vi "test b-field many sesnors tx ty derivatives.vi"() -> ()   [LabVIEW 2017]
uses:
  typedefs/magnet location tx ty.ctl
  typedefs/magnetomter reading set.ctl
panel:
  in  "magnet location tx ty BrV":T1={"x magnet"=20.0, "y magnet"=10.0, "z magnet"=100.0, "tx"=0.0, "ty"=0.0, "BrV"=-990.802948176856}
  out "size(s) 2":i32[](array[numeric])
  out "size(s)":i32[](array[numeric])
  out "derivatives":dbl[][](array[numeric]) format="%#_2p"
  out "numeric derivatives":dbl[][](array[numeric]) format="%#_2p"
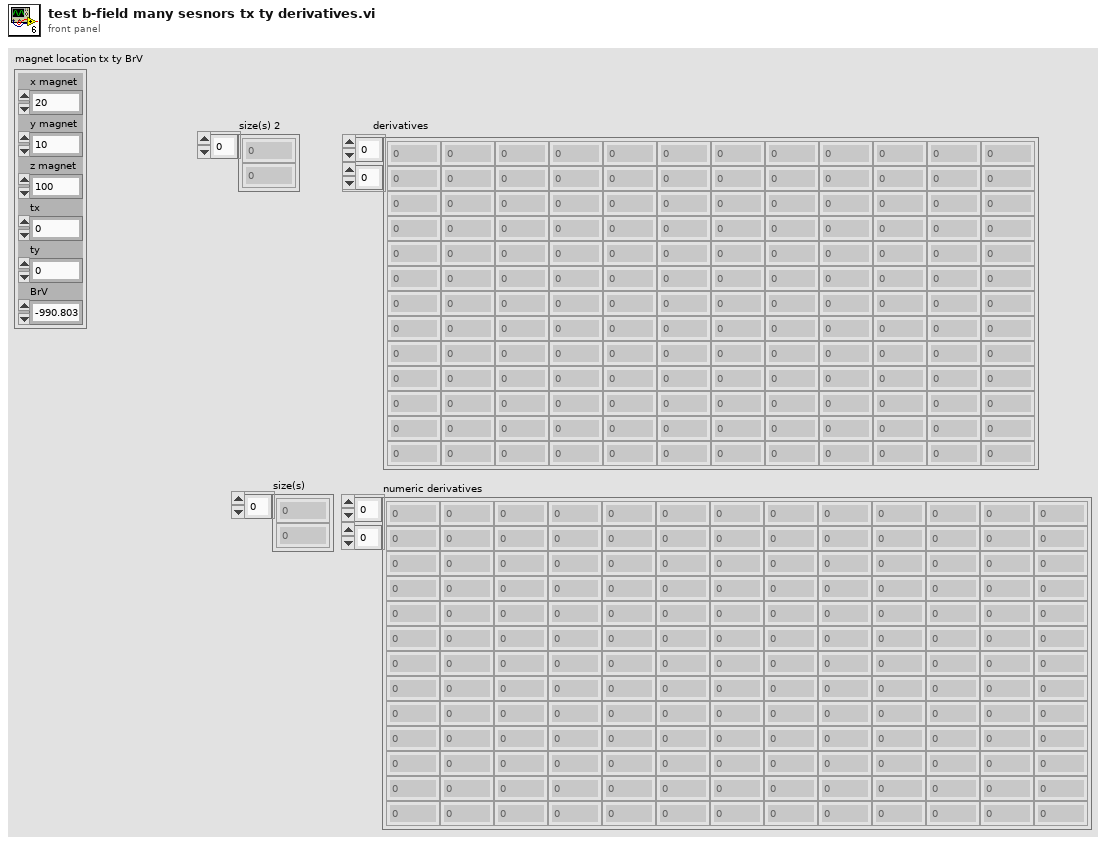
[diagram p1: front panel]
types:
  T1 = typedef "magnet location tx ty.ctl" = cluster{"x magnet":dbl, "y magnet":dbl, "z magnet":dbl, "tx":dbl, "ty":dbl, "BrV":dbl}
  T2 = typedef "magnetomter reading set.ctl" = cluster{"time":fxp<+,48,48>, "mag readings":cluster{"magnetometer index":dbl, "Bx":dbl, "By":dbl, "Bz":dbl, "magnetometer x":dbl, "magnetometer y":dbl}[]}
  T3 = cluster{"magnet location tx ty BrV[0]":dbl, "magnet location tx ty BrV[1]":dbl, "magnet location tx ty BrV[2]":dbl, "magnet location tx ty BrV[3]":dbl, "magnet location tx ty BrV[4]":dbl, "magnet location tx ty BrV[5]":dbl}
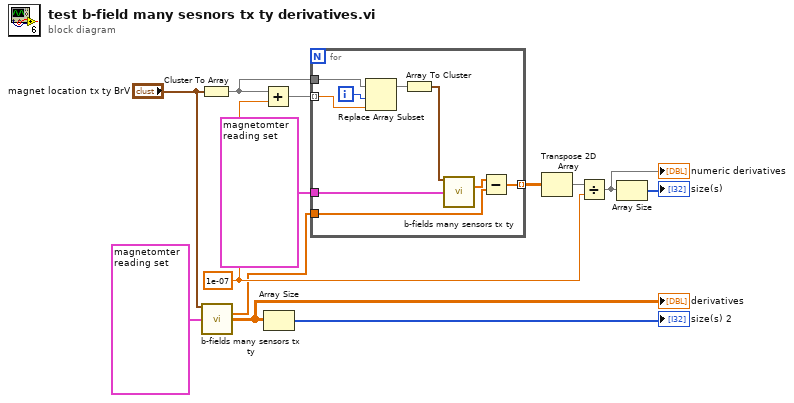
[diagram p0: block diagram]
diagram:
  w9 = 1e-07 ("y")
  n1 = Cluster To Array(cluster="magnet location tx ty BrV") -> (array=w12:dbl[])
  n2 = call "b-fields many sensors tx ty.vi"("magnet location tx ty BrV"="magnet location tx ty BrV", "Magnetometer reading set"=T2 {"time"=18872893554.0, "mag readings"=[{"magnetometer index"=0.0, "Bx"=-172.0634765625, "By"=-2.54296875, "Bz"=-1428.453125, "magnetometer x"=0.0, "magnetometer y"=0.0}, {"magnetometer index"=1.0, "Bx"=-208.375, "By"=357.4306640625, "Bz"=-182.794921875, "magnetometer x"=-22.5, "magnetometer y"=38.971}, {"magnetometer index"=2.0, "Bx"=-210.4453125, "By"=-333.25390625, "Bz"=-193.001953125, "magnetometer x"=-22.5, "magnetometer y"=-38.971}, {"magnetometer index"=3.0, "Bx"=467.15234375, "By"=36.216796875, "Bz"=-244.134765625, "magnetometer x"=45.0, "magnetometer y"=0.0}]}) -> ("pf - flat"=w1:dbl[], "derivative"=w2:dbl[][])  [unwired: 9 in, 3 out]
  "derivatives" <- w2
  n3 = Add(x=w12, y=w9) -> (x+y=w13:dbl[])
  n4 = Array Size(array=w2) -> (size(s)=→"size(s) 2":i32[])
  n5 = for {
    tunnel: w13 -> [w20] mode=indexing
    tunnel: w12 -> [w22]
    tunnel: T2 {"time"=18872893554.0, "mag readings"=[{"magnetometer index"=0.0, "Bx"=-172.0634765625, "By"=-2.54296875, "Bz"=-1428.453125, "magnetometer x"=0.0, "magnetometer y"=0.0}, {"magnetometer index"=1.0, "Bx"=-208.375, "By"=357.4306640625, "Bz"=-182.794921875, "magnetometer x"=-22.5, "magnetometer y"=38.971}, {"magnetometer index"=2.0, "Bx"=-210.4453125, "By"=-333.25390625, "Bz"=-193.001953125, "magnetometer x"=-22.5, "magnetometer y"=-38.971}, {"magnetometer index"=3.0, "Bx"=467.15234375, "By"=36.216796875, "Bz"=-244.134765625, "magnetometer x"=45.0, "magnetometer y"=0.0}]} ("magnetometer readings") -> [w17]
    tunnel: [w16] -> w10 mode=indexing
    tunnel: w1 -> [w15]
    i -> [w21]
    n6 = Replace Array Subset(array=w22, new element=w20, index=w21) -> (w19:dbl[])
    n7 = Array To Cluster(array=w19) -> (cluster=w18:T3)
    n8 = call "b-fields many sensors tx ty.vi"("magnet location tx ty BrV"=w18, "Magnetometer reading set"=w17) -> ("pf - flat"=w14:dbl[])  [unwired: 9 in, 4 out]
    n9 = Subtract(x=w14, y=w15) -> (x-y=w16:dbl[])
  }
  n10 = Transpose 2D Array(2D array=w10) -> (transposed array=w5:dbl[][])
  n11 = Divide(x=w5, y=w9) -> (x/y=w8:dbl[][])
  "numeric derivatives" <- w8
  n12 = Array Size(array=w8) -> (size(s)=→"size(s)":i32[])
